vi "ProcessFCCurrentsLE.vi"(9 "FC Data":waveform(dbl)[](array[waveform]), 10 "Bouncer Settings":T1 {"LE12C Voltage" format="%_4f"; "LE13C Voltage" format="%_4f"; "14C Voltage" format="%_4f"; "13C Voltage" format="%_4f"; "12C Voltage" format="%_4f"}, 11 "FC Offset":T2={"HE 12C Offset"=0.0, "HE 13CL Offset"=0.0, "HE 13CH Offset"=0.0, "LE FC Scale"=0, "HE C12 Scale"=0, "HE C13 Scale"=18} {"HE C13 Scale" items=["500 mA/V", "200 mA/V", "100 mA/V", "50 mA/V", "20 mA/V", "10 mA/V", "5 mA/V", "2 mA/V", "1 mA/V", "500 uA/V", "200 uA/V", "100 uA/V", "50 uA/V", "20 uA/V", "10 uA/V", "5 uA/V", "2 uA/V", "1 uA/V", "500 nA/V", "200 nA/V", "100 nA/V", "50 nA/V", "20 nA/V", "10 nA/V", "5 nA/V", "2 nA/V", "1 nA/V", "500 pA/V", "200 pA/V", "100 pA/V", "50 pA/V", "20 pA/V", "10 pA/V", "5 pA/V", "2 pA/V", "1 pA/V", ""]; "HE C12 Scale" items=["500 mA/V", "200 mA/V", "100 mA/V", "50 mA/V", "20 mA/V", "10 mA/V", "5 mA/V", "2 mA/V", "1 mA/V", "500 uA/V", "200 uA/V", "100 uA/V", "50 uA/V", "20 uA/V", "10 uA/V", "5 uA/V", "2 uA/V", "1 uA/V", "500 nA/V", "200 nA/V", "100 nA/V", "50 nA/V", "20 nA/V", "10 nA/V", "5 nA/V", "2 nA/V", "1 nA/V", "500 pA/V", "200 pA/V", "100 pA/V", "50 pA/V", "20 pA/V", "10 pA/V", "5 pA/V", "2 pA/V", "1 pA/V", ""]; "LE FC Scale" items=["500 mA/V", "200 mA/V", "100 mA/V", "50 mA/V", "20 mA/V", "10 mA/V", "5 mA/V", "2 mA/V", "1 mA/V", "500 uA/V", "200 uA/V", "100 uA/V", "50 uA/V", "20 uA/V", "10 uA/V", "5 uA/V", "2 uA/V", "1 uA/V", "500 nA/V", "200 nA/V", "100 nA/V", "50 nA/V", "20 nA/V", "10 nA/V", "5 nA/V", "2 nA/V", "1 nA/V", "500 pA/V", "200 pA/V", "100 pA/V", "50 pA/V", "20 pA/V", "10 pA/V", "5 pA/V", "2 pA/V", "1 pA/V", ""]}) -> (1 "Mean Currents":dbl[](array[numeric]), 2 "Output Waveforms":waveform(dbl)[](array[waveform]))   [LabVIEW 2013]
uses:
  ctl/FCOffset.ctl
  ctl/BouncerParameters.ctl
  <vilib>/Analysis/baseanly.llb/Mean (DBL).vi
  <vilib>/Waveform/WDTOps.llb/WDT Get Waveform Subset DBL (LV80).vi
  <vilib>/Analysis/NI_AALBase.lvlib
panel:
  out "Raw":waveform(dbl)[](graph)
  # "ms"
  # "us"
  # "kV"
  # "ms"
  # "us"
  # "kV"
  # "ms"
  # "us"
  # "kV"
  # "ms"
  # "us"
  # "kV"
  # "ms"
  # "us"
  # "kV"
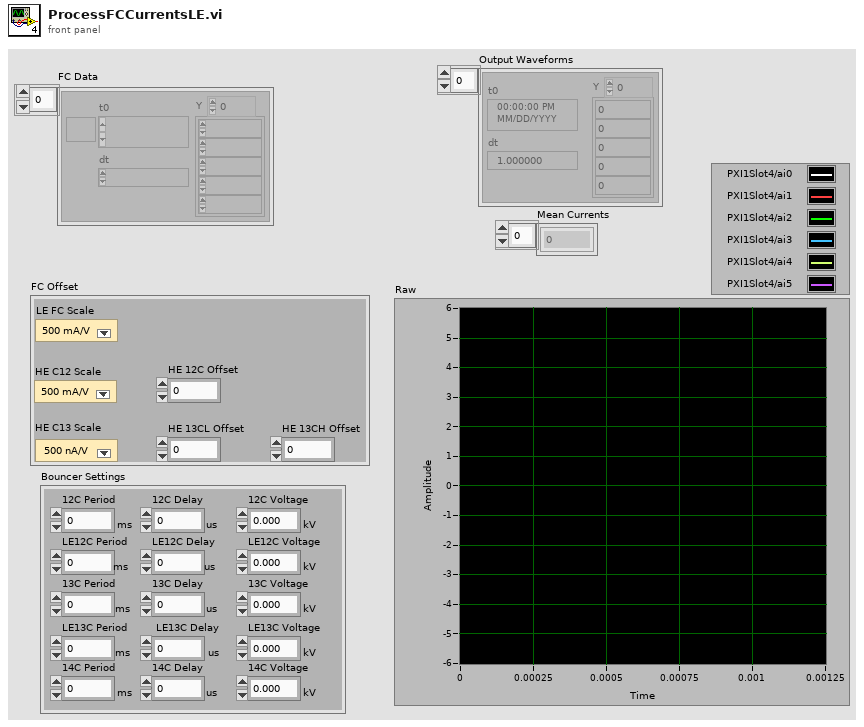
[diagram p1: front panel]
types:
  T1 = typedef "BouncerParameters.ctl" = cluster{"12C Period":dbl, "12C Delay":dbl, "12C Voltage":dbl, "13C Period":dbl, "13C Delay":dbl, "13C Voltage":dbl, "14C Period":dbl, "14C Delay":dbl, "14C Voltage":dbl, "LE13C Period":dbl, "LE13C Delay":dbl, "LE13C Voltage":dbl, "LE12C Period":dbl, "LE12C Delay":dbl, "LE12C Voltage":dbl}
  T2 = typedef "FCOffset.ctl" = cluster{"HE 12C Offset":dbl, "HE 13CL Offset":dbl, "HE 13CH Offset":dbl, "LE FC Scale":u16, "HE C12 Scale":u16, "HE C13 Scale":u16}
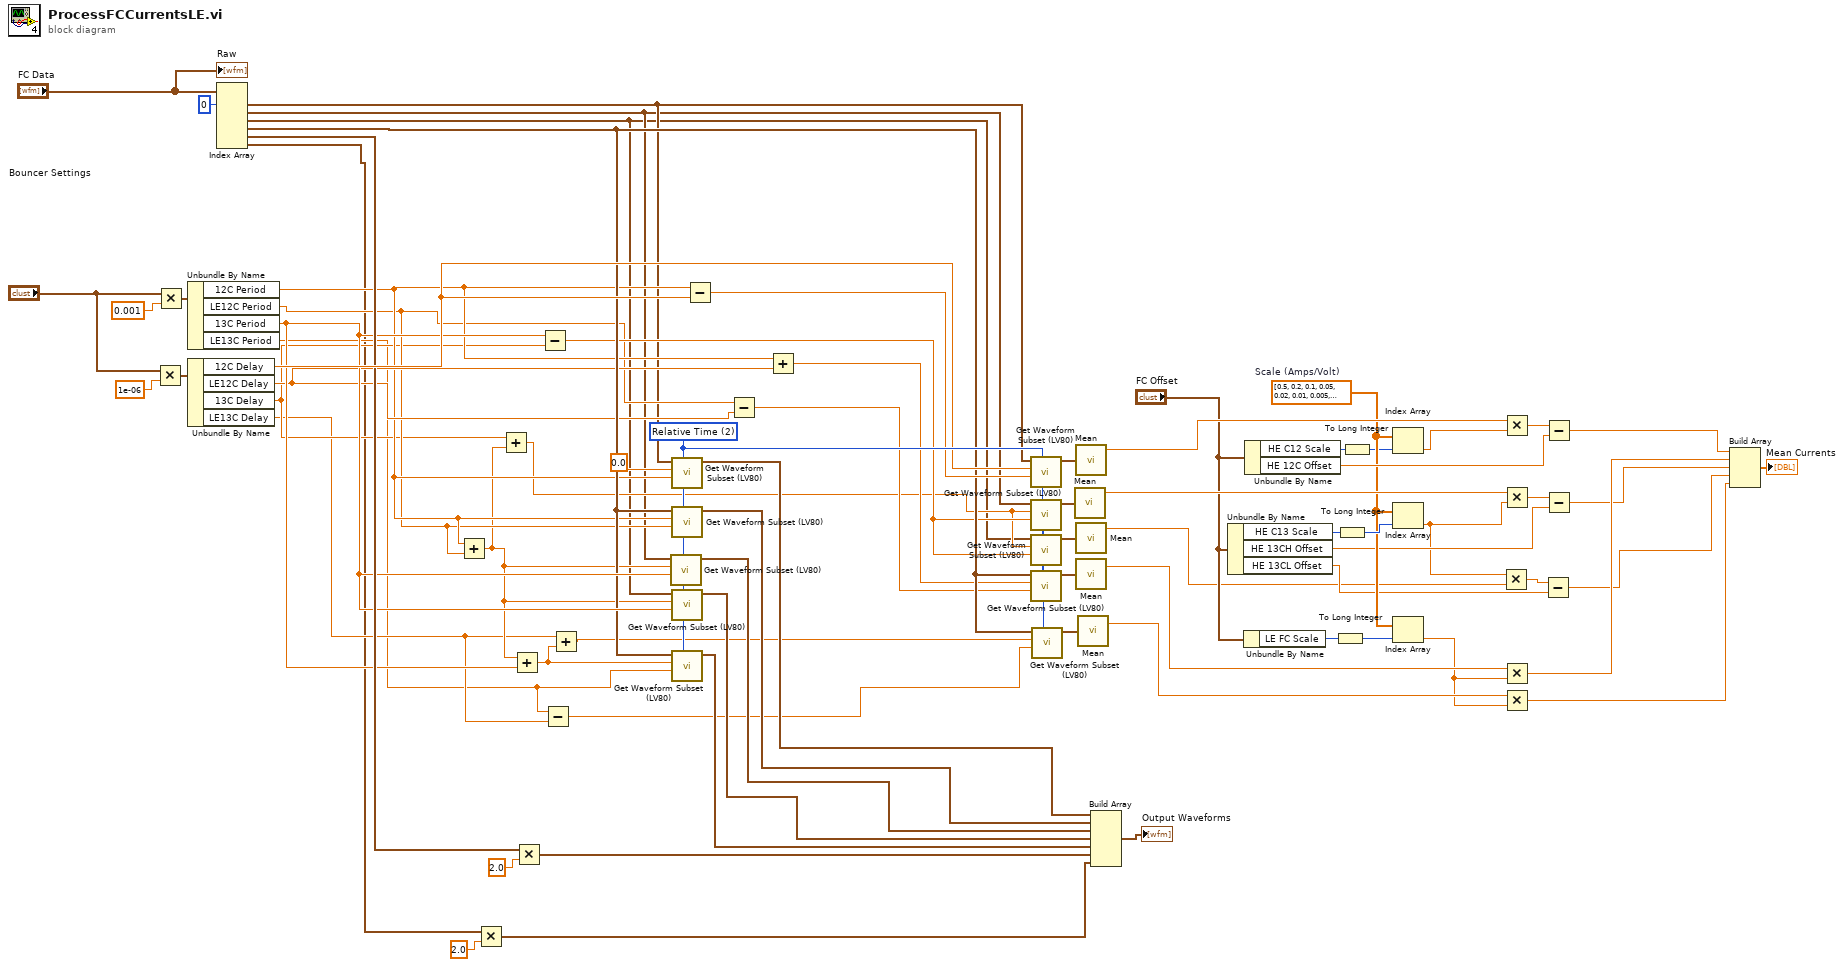
[diagram p0: block diagram]
diagram:
  w47 = dbl[] [0.5, 0.2, 0.1, 0.05, 0.02, 0.01, 0.005, 0.002, 0.001, 0.0005, 0.0002, 0.0001, 5e-05, 2e-05, 1e-05, 5e-06, 2e-06, 1e-06, 5e-07, 2e-07, 1e-07, 5e-08, 2e-08, 1e-08, 5e-09, 2e-09, 1e-09, 5e-10, 2e-10, 1e-10, 5e-11, 2e-11, 1e-11, 5e-12, 2e-12, 1e-12]  # Scale (Amps/Volt)
  w51 = u16 2 items=["Samples", "Absolute Time", "Relative Time"] ("start/duration format")
  n1 = Multiply(x="Bouncer Settings", y=1e-06) -> (x*y=w71:T1)
  n2 = Multiply(x="Bouncer Settings", y=0.001) -> (x*y=w73:T1)
  n3 = Unbundle By Name(w73) -> ("12C Period"=w17:dbl, "LE12C Period"=w16:dbl, "13C Period"=w36:dbl, "LE13C Period"=w9:dbl)
  n4 = Unbundle By Name(w71) -> ("12C Delay"=w43:dbl, "LE12C Delay"=w19:dbl, "13C Delay"=w14:dbl, "LE13C Delay"=w10:dbl)
  n5 = Index Array(array="FC Data", index #1=0 ("index")) -> (element #1=w7:waveform(dbl), element #2=w6:waveform(dbl), element #3=w5:waveform(dbl), element #4=w24:waveform(dbl), element #5=w40:waveform(dbl), element #6=w1:waveform(dbl))  [unwired: 5 in]
  n6 = Add(x=w17, y=w16) -> (x+y=w15:dbl)
  n7 = Multiply(x=w1, y=2.0) -> (x*y=w2:waveform(dbl))
  n8 = Add(x=w14, y=w15) -> (x+y=w13:dbl)
  n9 = Add(x=w15, y=w36) -> (x+y=w12:dbl)
  n10 = Multiply(x=w40, y=2.0) -> (x*y=w45:waveform(dbl))
  n11 = Subtract(x=w36, y=w14) -> (x-y=w23:dbl)
  n12 = Subtract(x=w9, y=w10) -> (x-y=w8:dbl)
  n13 = Add(x=w10, y=w12) -> (x+y=w11:dbl)
  n14 = call-poly <vilib>:"Get Waveform Subset (LV80).vi"("start/duration format"=w51, "duration"=w36, "start samples/time"=w15, "waveform in"=w6) -> ("waveform out"=w27:waveform(dbl))  [unwired: 1 in, 4 out]
  n15 = call-poly <vilib>:"Get Waveform Subset (LV80).vi"("start/duration format"=w51, "duration"=w17, "start samples/time"=0.0, "waveform in"=w7) -> ("waveform out"=w25:waveform(dbl))  [unwired: 1 in, 4 out]
  n16 = call-poly <vilib>:"Get Waveform Subset (LV80).vi"("start/duration format"=w51, "duration"=w16, "start samples/time"=w17, "waveform in"=w24) -> ("waveform out"=w26:waveform(dbl))  [unwired: 1 in, 4 out]
  n17 = call-poly <vilib>:"Get Waveform Subset (LV80).vi"("start/duration format"=w51, "duration"=w36, "start samples/time"=w15, "waveform in"=w5) -> ("waveform out"=w22:waveform(dbl))  [unwired: 1 in, 4 out]
  n18 = call-poly <vilib>:"Get Waveform Subset (LV80).vi"("start/duration format"=w51, "duration"=w9, "start samples/time"=w12, "waveform in"=w24) -> ("waveform out"=w39:waveform(dbl))  [unwired: 1 in, 4 out]
  n19 = Subtract(x=w17, y=w43) -> (x-y=w42:dbl)
  n20 = Subtract(x=w16, y=w19) -> (x-y=w18:dbl)
  n21 = Add(x=w17, y=w19) -> (x+y=w20:dbl)
  n22 = call-poly <vilib>:"Get Waveform Subset (LV80).vi"("start/duration format"=w51, "duration"=w42, "start samples/time"=w43, "waveform in"=w7) -> ("waveform out"=w69:waveform(dbl))  [unwired: 1 in, 4 out]
  n23 = call-poly <vilib>:"Get Waveform Subset (LV80).vi"("start/duration format"=w51, "duration"=w23, "start samples/time"=w13, "waveform in"=w6) -> ("waveform out"=w67:waveform(dbl))  [unwired: 1 in, 4 out]
  n24 = call-poly <vilib>:"Get Waveform Subset (LV80).vi"("start/duration format"=w51, "duration"=w23, "start samples/time"=w13, "waveform in"=w5) -> ("waveform out"=w50:waveform(dbl))  [unwired: 1 in, 4 out]
  n25 = call-poly <vilib>:"Get Waveform Subset (LV80).vi"("start/duration format"=w51, "duration"=w18, "start samples/time"=w20, "waveform in"=w24) -> ("waveform out"=w66:waveform(dbl))  [unwired: 1 in, 4 out]
  n26 = call-poly <vilib>:"Get Waveform Subset (LV80).vi"("start/duration format"=w51, "duration"=w8, "start samples/time"=w11, "waveform in"=w24) -> ("waveform out"=w68:waveform(dbl))  [unwired: 1 in, 4 out]
  n27 = call-poly <vilib>:"Mean.vi"("X"=w67) -> ("mean"=w64:dbl)  [unwired: 1 out]
  n28 = call-poly <vilib>:"Mean.vi"("X"=w69) -> ("mean"=w65:dbl)  [unwired: 1 out]
  n29 = call-poly <vilib>:"Mean.vi"("X"=w50) -> ("mean"=w21:dbl)  [unwired: 1 out]
  n30 = call-poly <vilib>:"Mean.vi"("X"=w66) -> ("mean"=w38:dbl)  [unwired: 1 out]
  n31 = call-poly <vilib>:"Mean.vi"("X"=w68) -> ("mean"=w37:dbl)  [unwired: 1 out]
  n32 = Build Array(w25, w26, w27, w22, w39, w45, w2) -> (→"Output Waveforms":waveform(dbl)[])
  n33 = Unbundle By Name("FC Offset") -> ("HE C13 Scale"=w63:u16, "HE 13CH Offset"=w33:dbl, "HE 13CL Offset"=w29:dbl)
  n34 = Unbundle By Name("FC Offset") -> ("LE FC Scale"=w32:u16)
  n35 = Unbundle By Name("FC Offset") -> ("HE C12 Scale"=w35:u16, "HE 12C Offset"=w60:dbl)
  n36 = To Long Integer(number=w32) -> (32bit integer=w31:i32)
  n37 = To Long Integer(number=w63) -> (32bit integer=w59:i32)
  n38 = To Long Integer(number=w35) -> (32bit integer=w34:i32)
  n39 = Index Array(array=w47, index=w34) -> (element=w41:dbl)
  n40 = Index Array(array=w47, index=w59) -> (element=w28:dbl)
  n41 = Index Array(array=w47, index=w31) -> (element=w30:dbl)
  n42 = Multiply(x=w28, y=w21) -> (x*y=w49:dbl)
  n43 = Multiply(x=w65, y=w41) -> (x*y=w62:dbl)
  n44 = Multiply(x=w64, y=w28) -> (x*y=w61:dbl)
  n45 = Multiply(x=w38, y=w30) -> (x*y=w55:dbl)
  n46 = Multiply(x=w37, y=w30) -> (x*y=w53:dbl)
  n47 = Subtract(x=w49, y=w29) -> (x-y=w48:dbl)
  n48 = Subtract(x=w62, y=w60) -> (x-y=w56:dbl)
  n49 = Subtract(x=w61, y=w33) -> (x-y=w54:dbl)
  n50 = Build Array(w56, w55, w54, w48, w53) -> (→"Mean Currents":dbl[])
  "Raw" <- "FC Data"
